vi "MicTest_trrs.vi"() -> ()   [LabVIEW 2014]
uses:
  <vilib>/eio/EIONode/EIONode.xnode
  <vilib>/rvi/eio/common/nirviEmuTemplateMethod_errors.vi
panel:
  out "data":dynamicdata(graph)
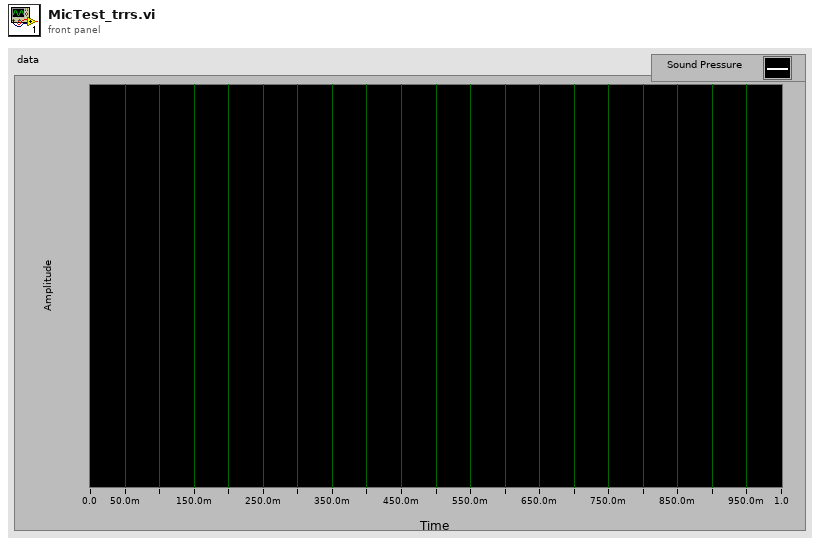
[diagram p1: front panel]
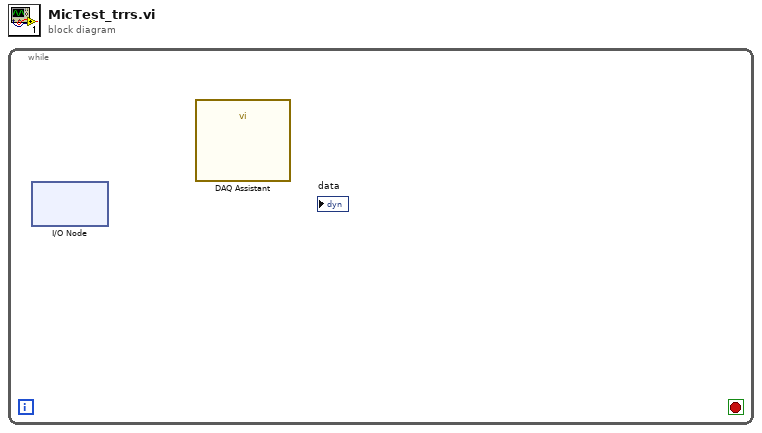
[diagram p0: block diagram]
diagram:
  n1 = while {
    stop <- _ stop-if-true
    n2 = xnode "I/O Node"() -> ()  [unwired: 1 in, 2 out]
    n3 = call "DAQ Assistant"() -> ()  [unwired: 12 in]
  }
